vi "error and results.vi"() -> ()   [LabVIEW 2016]
uses:
  controls/cycle results control.ctl
  controls/unique results control.ctl
  controls/error calculations.ctl
panel:
  out "cycle error":dbl[][](array[numeric])
  out "cycle result":dbl[](array[numeric])
  out "cycle external error":dbl[](array[numeric])
  in  "Charge State":dbl=3.0
  out "cycle internal error":dbl[](array[numeric])
  out "cycle results":T1 {"cycle results dbl" format="%#_6f"}
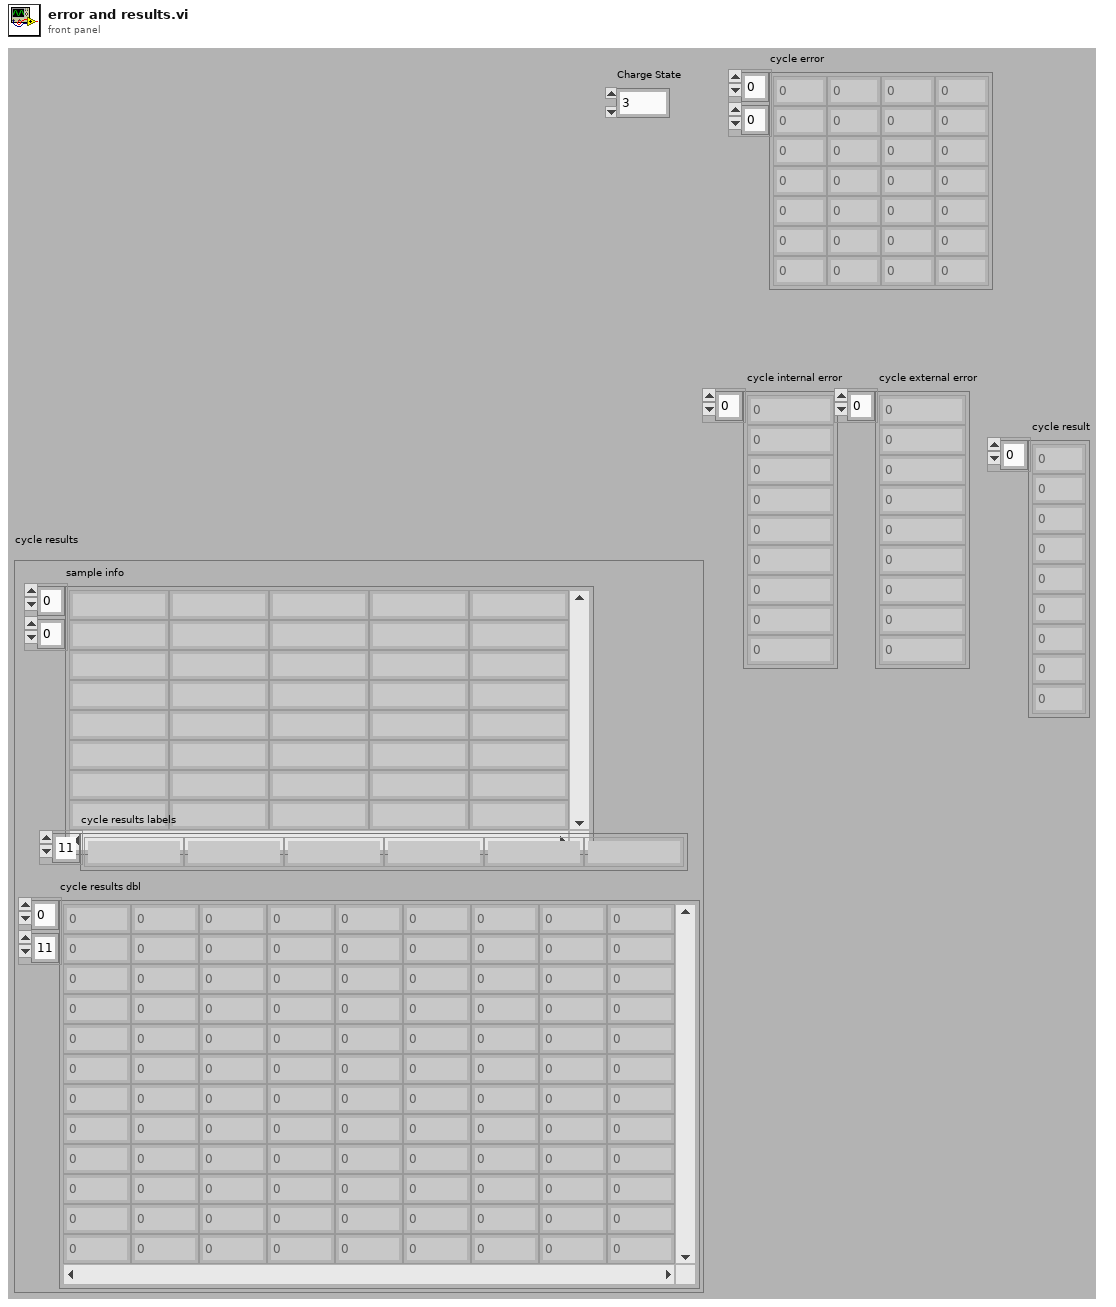
[diagram p1: front panel]
types:
  T1 = typedef "cycle results control.ctl" = cluster{"sample info":string[][], "cycle results labels":string[], "cycle results dbl":dbl[][]}
  T2 = typedef "error calculations.ctl" = string
  T3 = typedef "unique results control.ctl" = string
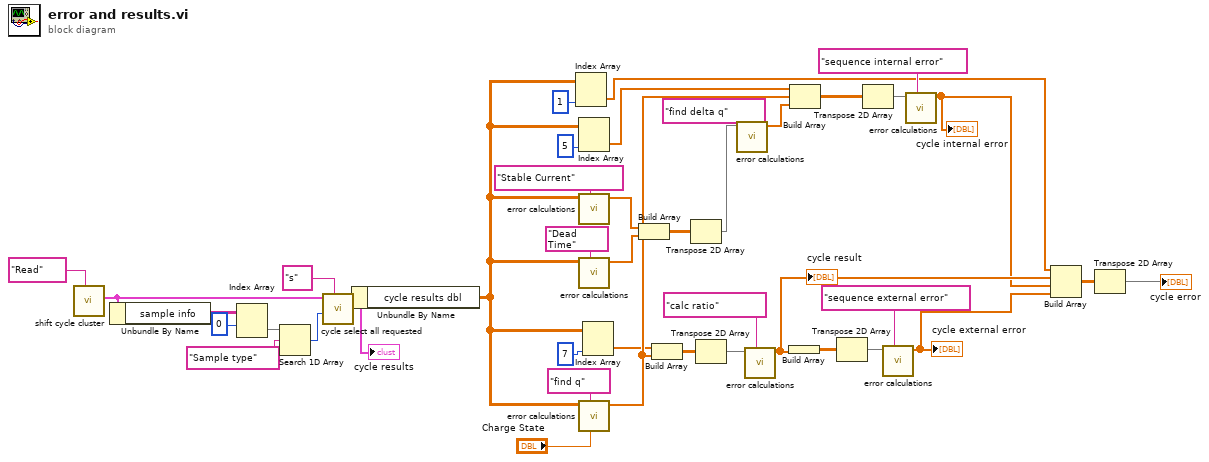
[diagram p0: block diagram]
diagram:
  n1 = call "shift cycle cluster.vi"("read write shift"="Read") -> ("cycle results cluster out"=w1:T1)  [unwired: 9 in, 1 out]
  n2 = Unbundle By Name(w1) -> ("sample info"=w41:string[][])
  n3 = Index Array(array=w41, index (row)=0) -> (element=w39:string[])  [unwired: 1 in]
  n4 = Search 1D Array(1D array=w39, element="Sample type") -> (index of element=w37:i32)  [unwired: 1 in]
  n5 = call "cycle select all requested.vi"("which value to be selected"=T3 "s", "value that will be sorted In"=w37, "cycle results cluster IN"=w1) -> ("cycle results cluster out"=w35:T1)  [unwired: 7 in, 1 out]
  "cycle results" <- w35
  n6 = Unbundle By Name(w35) -> ("cycle results dbl"=w10:dbl[][])
  n7 = Index Array(array=w10, index (col)=1 ("disabled index (col)")) -> (element=w8:dbl[])  [unwired: 1 in]
  n8 = Index Array(array=w10, index (col)=5) -> (element=w12:dbl[])  [unwired: 1 in]
  n9 = call "error calculations.vi"("Error calculation"=T2 "Stable Current", "cycle results dbl"=w10) -> ("array out"=w32:dbl[])  [unwired: 8 in, 1 out]
  n10 = call "error calculations.vi"("Error calculation"=T2 "Dead Time", "cycle results dbl"=w10) -> ("array out"=w31:dbl[])  [unwired: 8 in, 1 out]
  n11 = call "error calculations.vi"("Charge State"="Charge State", "Error calculation"=T2 "find q", "cycle results dbl"=w10) -> ("array out"=w21:dbl[])  [unwired: 7 in, 1 out]
  n12 = Index Array(array=w10, index (col)=7) -> (element=w14:dbl[])  [unwired: 1 in]
  n13 = Build Array(w32, w31) -> (w30:dbl[][])
  n14 = Build Array(w14, w21) -> (w25:dbl[][])
  n15 = Transpose 2D Array(2D array=w30) -> (transposed array=w28:dbl[][])
  n16 = Transpose 2D Array(2D array=w25) -> (transposed array=w22:dbl[][])
  n17 = call "error calculations.vi"("Error calculation"=T2 "find delta q", "cycle results dbl"=w28) -> ("array out"=w19:dbl[])  [unwired: 8 in, 1 out]
  n18 = call "error calculations.vi"("Error calculation"=T2 "calc ratio", "cycle results dbl"=w22) -> ("array out"=w7:dbl[])  [unwired: 8 in, 1 out]
  "cycle result" <- w7
  n19 = Build Array(w7) -> (w17:dbl[][])
  n20 = Build Array(w12, w21, w19) -> (w20:dbl[][])
  n21 = Transpose 2D Array(2D array=w17) -> (transposed array=w16:dbl[][])
  n22 = Transpose 2D Array(2D array=w20) -> (transposed array=w18:dbl[][])
  n23 = call "error calculations.vi"("Error calculation"=T2 "sequence external error", "cycle results dbl"=w16) -> ("array out"=w5:dbl[])  [unwired: 8 in, 1 out]
  "cycle external error" <- w5
  n24 = call "error calculations.vi"("Error calculation"=T2 "sequence internal error", "cycle results dbl"=w18) -> ("array out"=w6:dbl[])  [unwired: 8 in, 1 out]
  "cycle internal error" <- w6
  n25 = Build Array(w8, w7, w6, w5) -> (w4:dbl[][])
  n26 = Transpose 2D Array(2D array=w4) -> (transposed array=→"cycle error":dbl[][])
